vi "Find FPGA Addon Custom Devices.vi"(8 "error in (no error)":errorcluster, 11 "target in":refnum<k24>) -> (0 "error out":errorcluster, 1 "found ?":bool, 2 "fpga addon refnums out":T1[](array[typedef]) format="%.0x", 3 "target out":refnum<k24>)   [LabVIEW 2018, in "Scripting API.lvlib"]
uses:
  Scripting API.lvlib
  NationalInstruments.VeriStand.SystemDefinitionAPI
  <vilib>/NI Veristand/Custom Device API/Custom Device Item Ref.ctl
  <vilib>/NI Veristand/Custom Device API/Custom Device API.lvlib
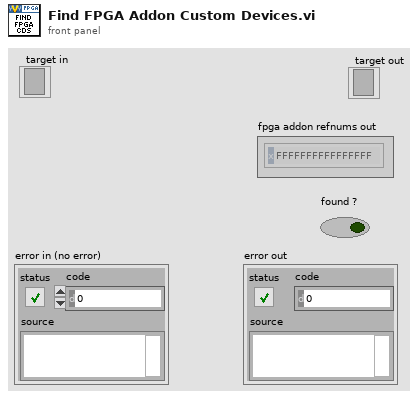
[diagram p1: front panel]
types:
  T1 = typedef "Custom Device API.lvlib/Custom Device Item Ref.ctl" = u64
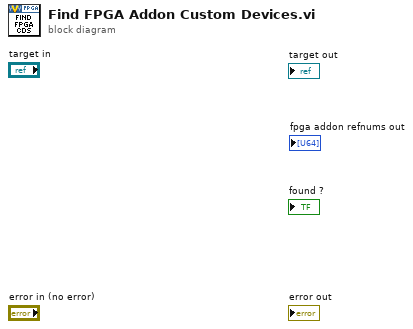
[diagram p0: block diagram]
diagram:
